vi "subAcquisition_AcquirngColor.vi"(7 "Bool Refnum":refnum<vi>, 11 "Filter Set":i32(ring) items=["R-QuasAr", "R-Cy5", "R-mCherry", "R-mOrange", "R-GFP", "R-CFP/DAPI", "R-BFP", "R-LED", "SDC-Cy5", "SDC-mCherry", "SDC-mO2", "SDC-GFP", "SDC-CFP/DAPI", "SDC-BFP", "SDC-LED"]) -> ()   [LabVIEW 2015]
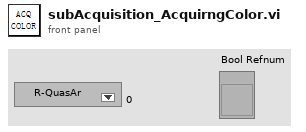
[diagram p1: front panel]
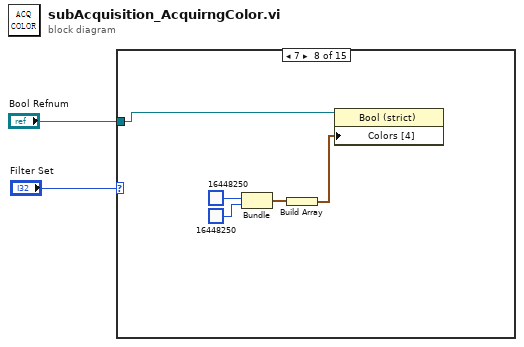
[diagram p0: block diagram]
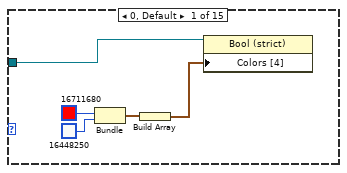
[diagram p2: hidden frame]
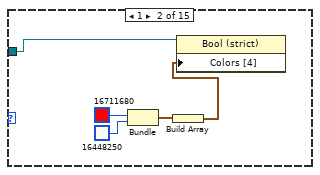
[diagram p3: hidden frame]
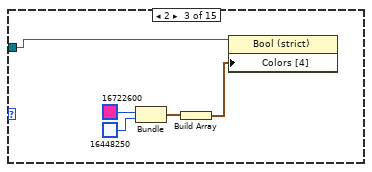
[diagram p4: hidden frame]
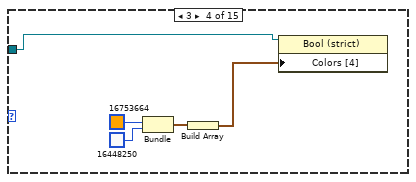
[diagram p5: hidden frame]
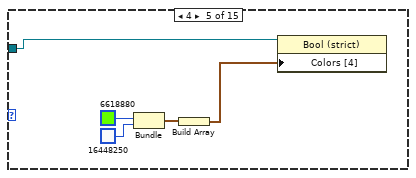
[diagram p6: hidden frame]
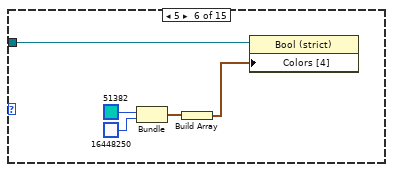
[diagram p7: hidden frame]
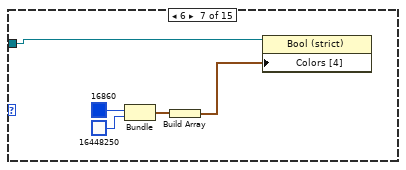
[diagram p8: hidden frame]
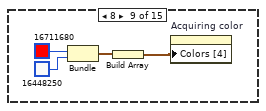
[diagram p9: hidden frame]
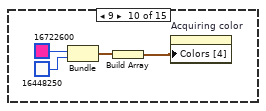
[diagram p10: hidden frame]
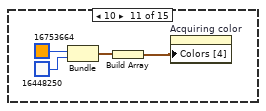
[diagram p11: hidden frame]
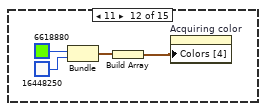
[diagram p12: hidden frame]
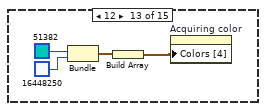
[diagram p13: hidden frame]
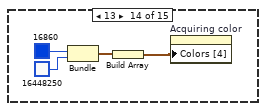
[diagram p14: hidden frame]
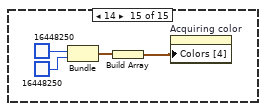
[diagram p15: hidden frame]
diagram:
  n1 = case shown="7" "Filter Set" {
    tunnel: "Bool Refnum" -> [w4 w9 w14 w19 w24 w29 w34 w39 _ _ _ _ _ _ _]
    frame 0, Default {
      n2 = Bundle(u32 16711680, u32 16448250) -> (w6:cluster{u32, u32})  [unwired: 1 in]
      n3 = Build Array(w6) -> (w3:cluster{u32, u32}[])
      n4 = property class="Bool (strict)"(reference=w4, "Colors [4]"=w3) -> ()  [unwired: 1 in, 2 out]
    }
    frame 1 {
      n5 = Bundle(u32 16711680, u32 16448250) -> (w11:cluster{u32, u32})  [unwired: 1 in]
      n6 = Build Array(w11) -> (w8:cluster{u32, u32}[])
      n7 = property class="Bool (strict)"(reference=w9, "Colors [4]"=w8) -> ()  [unwired: 1 in, 2 out]
    }
    frame 2 {
      n8 = Bundle(u32 16722600, u32 16448250) -> (w16:cluster{u32, u32})  [unwired: 1 in]
      n9 = Build Array(w16) -> (w13:cluster{u32, u32}[])
      n10 = property class="Bool (strict)"(reference=w14, "Colors [4]"=w13) -> ()  [unwired: 1 in, 2 out]
    }
    frame 3 {
      n11 = Bundle(u32 16753664, u32 16448250) -> (w21:cluster{u32, u32})  [unwired: 1 in]
      n12 = Build Array(w21) -> (w18:cluster{u32, u32}[])
      n13 = property class="Bool (strict)"(reference=w19, "Colors [4]"=w18) -> ()  [unwired: 1 in, 2 out]
    }
    frame 4 {
      n14 = Bundle(u32 6618880, u32 16448250) -> (w26:cluster{u32, u32})  [unwired: 1 in]
      n15 = Build Array(w26) -> (w23:cluster{u32, u32}[])
      n16 = property class="Bool (strict)"(reference=w24, "Colors [4]"=w23) -> ()  [unwired: 1 in, 2 out]
    }
    frame 5 {
      n17 = Bundle(u32 51382, u32 16448250) -> (w31:cluster{u32, u32})  [unwired: 1 in]
      n18 = Build Array(w31) -> (w28:cluster{u32, u32}[])
      n19 = property class="Bool (strict)"(reference=w29, "Colors [4]"=w28) -> ()  [unwired: 1 in, 2 out]
    }
    frame 6 {
      n20 = Bundle(u32 16860, u32 16448250) -> (w36:cluster{u32, u32})  [unwired: 1 in]
      n21 = Build Array(w36) -> (w33:cluster{u32, u32}[])
      n22 = property class="Bool (strict)"(reference=w34, "Colors [4]"=w33) -> ()  [unwired: 1 in, 2 out]
    }
    frame 7 {
      n23 = Bundle(u32 16448250, u32 16448250) -> (w41:cluster{u32, u32})  [unwired: 1 in]
      n24 = Build Array(w41) -> (w38:cluster{u32, u32}[])
      n25 = property class="Bool (strict)"(reference=w39, "Colors [4]"=w38) -> ()  [unwired: 1 in, 2 out]
    }
    frame 8 {
      n26 = Bundle(u32 16711680, u32 16448250) -> (w45:cluster{u32, u32})  [unwired: 1 in]
      n27 = Build Array(w45) -> (w43:cluster{u32, u32}[])
      n28 = property on="Acquiring color" class="Bool (strict)"("Colors [4]"=w43) -> ()  [unwired: 2 in, 2 out]
    }
    frame 9 {
      n29 = Bundle(u32 16722600, u32 16448250) -> (w49:cluster{u32, u32})  [unwired: 1 in]
      n30 = Build Array(w49) -> (w47:cluster{u32, u32}[])
      n31 = property on="Acquiring color" class="Bool (strict)"("Colors [4]"=w47) -> ()  [unwired: 2 in, 2 out]
    }
    frame 10 {
      n32 = Bundle(u32 16753664, u32 16448250) -> (w53:cluster{u32, u32})  [unwired: 1 in]
      n33 = Build Array(w53) -> (w51:cluster{u32, u32}[])
      n34 = property on="Acquiring color" class="Bool (strict)"("Colors [4]"=w51) -> ()  [unwired: 2 in, 2 out]
    }
    frame 11 {
      n35 = Bundle(u32 6618880, u32 16448250) -> (w57:cluster{u32, u32})  [unwired: 1 in]
      n36 = Build Array(w57) -> (w55:cluster{u32, u32}[])
      n37 = property on="Acquiring color" class="Bool (strict)"("Colors [4]"=w55) -> ()  [unwired: 2 in, 2 out]
    }
    frame 12 {
      n38 = Bundle(u32 51382, u32 16448250) -> (w61:cluster{u32, u32})  [unwired: 1 in]
      n39 = Build Array(w61) -> (w59:cluster{u32, u32}[])
      n40 = property on="Acquiring color" class="Bool (strict)"("Colors [4]"=w59) -> ()  [unwired: 2 in, 2 out]
    }
    frame 13 {
      n41 = Bundle(u32 16860, u32 16448250) -> (w65:cluster{u32, u32})  [unwired: 1 in]
      n42 = Build Array(w65) -> (w63:cluster{u32, u32}[])
      n43 = property on="Acquiring color" class="Bool (strict)"("Colors [4]"=w63) -> ()  [unwired: 2 in, 2 out]
    }
    frame 14 {
      n44 = Bundle(u32 16448250, u32 16448250) -> (w69:cluster{u32, u32})  [unwired: 1 in]
      n45 = Build Array(w69) -> (w67:cluster{u32, u32}[])
      n46 = property on="Acquiring color" class="Bool (strict)"("Colors [4]"=w67) -> ()  [unwired: 2 in, 2 out]
    }
  }
